vi "Fpga-FPGANic-Top.vi"() -> ()   [LabVIEW 2018]
uses:
  <instrlib>/_niInstr/Network/Ethernet/MAC/CLIP/v1/Resources.ctl
  <vilib>/Platform/TimedLoop/XDataNode/timing_clust.ctl
  <vilib>/Platform/TimedLoop/XDataNode/nitl_modes.ctl
  <vilib>/Platform/TimedLoop/XDataNode/wakeup.ctl
  States/FPGANic.Read.States.ctl
  <instrlib>/_niInstr/Network/Ethernet/MAC/Raw Stream/v1/niInstr Ethernet MAC Raw Stream v1.lvclass
  <instrlib>/_niInstr/Network/Ethernet/Utility/v1/FPGA/Network Data Stream.ctl
  States/FPGANic.Write.States.ctl
  <vilib>/rvi/Emulation/niFpgaSctlEmulationGetInTimedLoop.vi
  <vilib>/rvi/Emulation/niFpgaEmulationReportErrorSimple.vi
  <vilib>/rvi/Emulation/niFpgaGetClockAttributes.vi
  <vilib>/rvi/Emulation/niFpgaCriticalErrorInLSC.vi
  <vilib>/rvi/eio/common/nirviEmuTemplateMethod_errors.vi
  <vilib>/rvi/interface/RandomDataEmulation/niFpgaRandomDataHandleErrors.vi
  <vilib>/rvi/DataTransferAndStorage/Container/Common/niFpgaContainerGetUniqueNameForEmu.vi
  <vilib>/rvi/DataTransferAndStorage/Container/Common/niFpgaContainerSetEmuInfo.vi
  <vilib>/rvi/eio/common/nirviEmuReportErrorAndStop.vi
  <vilib>/rvi/DataTransferAndStorage/Container/Common/niFpgaContainerExecOnDevCompGetState.vi
  <vilib>/rvi/Emulation/niFpgaEmulationIsFPGAContextNoSignature.vi
  <vilib>/rvi/errors/niFpgaSetErrorForExecOnDevCompSimple.vi
  <vilib>/rvi/FIFO/Fifo_Resource/nirvififoEmulationSetSize.vi
  <vilib>/rvi/FIFO/Fifo_Resource/nirviFifoEmulationQueueMgr.vi
  <instcachedir>/0/nirviFifoEmulationQueueMgr_E5CAEC123FF24DC58D834DCA3CDAA9B5.lvgen/nirviFifoEmulationQueueMgr_E5CAEC123FF24DC58D834DCA3CDAA9B5_003.vi
  <vilib>/rvi/FIFO/Fifo_Resource/nirvififoEmulationDetermineInputValidOut.vi
  <vilib>/rvi/FIFO/Fifo_Resource/nirvififoEmulationCreateLock.vi
  <vilib>/rvi/Emulation/niFpgaProcessEmulError.vi
  <vilib>/rvi/FIFO/Fifo_Resource/nirvififoEmulationObtainLock.vi
  <vilib>/rvi/FIFO/Fifo_Resource/nirvififoEmulationReleaseLock.vi
  <vilib>/rvi/occurrence/nirviWaitOnOccurrenceBase.vi
  <vilib>/rvi/errors/nirviReportUnexpectedCaseInternalError.vi
  <vilib>/rvi/errors/nirviReportUnexpectedCaseInternalError (U32).vi
  <vilib>/Utility/error.llb/Clear Errors.vi
  <instrlib>/_niInstr/Network/Ethernet/MAC/Raw Stream/v1/Read End of Bad Frame.vi
  <instrlib>/_niInstr/Network/Ethernet/MAC/Raw Stream/v1/Read End of Good Frame.vi
  <instrlib>/_niInstr/Network/Ethernet/MAC/Raw Stream/v1/Read Data Stream.vi
  <instrlib>/_niInstr/Network/Ethernet/MAC/Raw Stream/v1/Write Data Stream.vi
  <instrlib>/_niInstr/Network/Ethernet/MAC/Raw Stream/v1/Write End of Good Frame.vi
  <vilib>/Platform/TimedLoop/XDataNode/XDataNode.xnode
  <vilib>/eio/EIONode/EIONode.xnode
  <vilib>/rvi/DataTransferAndStorage/Container/XNode/niFpgaContainer.xnode
  <vilib>/rvi/interface/RandomDataEmulation/nirviRandomDataFpgaReadWriteTemplate.vi
  <vilib>/rvi/LocalResourceManager/LocalResourceManager.xnode
  <vilib>/rvi/FIFO/Fifo_Resource/niFpgaFifoEmulationRefIn.vi
  <instrlib>/_niInstr/Network/Ethernet/MAC/CLIP/v1/niInstr Ethernet MAC - CLIP v1.lvclass
  <vilib>/Platform/TimedLoop/XDataNode/XDNodeRunTimeDep.lvlib
  <instrlib>/_niInstr/Network/Ethernet/Utility/v1/FPGA/niInstr Ethernet Utilities FPGA v1.lvlib
panel:
  in  "Zero-out":bool
  in  "Flip_in":bool
  in  "d_microblaze_i\\reset_rtl":bool=TRUE
  out "GPIO #1 out":u32
  in  "GPIO #1 in":u32
  in  "d_microblaze_i\\AXI_STR_RXD_3_tkeep":u8=15
  out "mgtrefclks_locked":bool
  out "mgtrefclks_valid":bool
  out "posc_complete":bool
  out "sPort0_Power_Good":bool
  out "sPort1_Power_Good":bool
  out "signal_detect_Port0":bool
  out "signal_detect_Port1":bool
  out "aBlockLockPort0":bool
  out "aBlockLockPort1":bool
  out "GPIO #2 out":u32
  in  "GPIO #2 in":u32
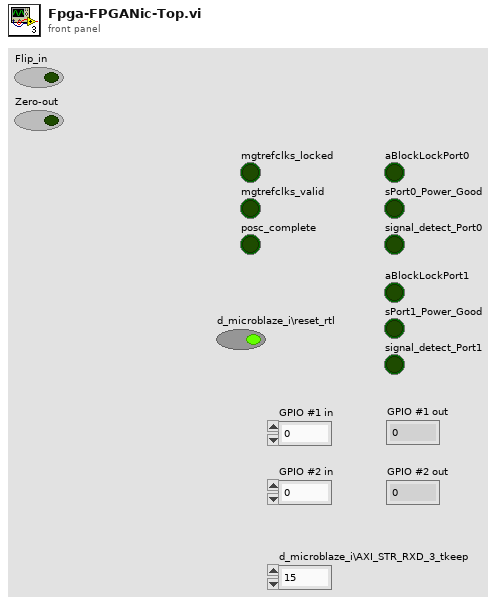
[diagram p1: front panel]
types:
  T1 = typedef "niInstr Ethernet MAC - CLIP v1.lvclass/Resources.ctl" = cluster{"RX":cluster{"TData":refnum<k21>, "TValid":refnum<k21>, "TKeep":refnum<k21>, "TLast":refnum<k21>, "TUser":refnum<k21>}, "TX":cluster{"TData":refnum<k21>, "TValid":refnum<k21>, "TKeep":refnum<k21>, "TLast":refnum<k21>, "TReady":refnum<k21>}, "Pause resources":cluster{"cPauseValuePort":refnum<k21>, "cPauseReqPort":refnum<k21>}, "MAC Clock":refnum<k21>}
  T2 = typedef "XDNodeRunTimeDep.lvlib/timing_clust.ctl" = cluster{"Expected End [f-1]":u64, "Actual End [f-1]":u64, "Finished Late? [f-1]":bool, "Expected End [i-1]":u64, "Actual End [i-1]":u64, "Finished Late? [i-1]":bool, "Expected Start [i]":u64, "Actual Start [i]":u64, "Expected Start [f]":u64, "Actual Start [f]":u64, "Source Name":string, "Structure Name":string, "Period":i64, "Deadline":i64, "Offset":i64, "Start":i64, "Priority":i32, "Timeout":i32, "Mode":T3, "Wakeup Reason":T4, "Error":errorcluster, "Source Type":string, "Secondary Source Type":string, "Global End Time":u64, "Global Start Time":u64, "Frame Duration":u64, "Iteration Duration":u64, "Assigned CPU":i32, "I/O Scan Engine Mode":u32}
  T3 = typedef "XDNodeRunTimeDep.lvlib/nitl_modes.ctl" = enum32{"No Change", "Process missed periods, maintain original phase", "Discard missed periods, maintain original phase", "Process missed periods, ignore original phase", "Discard missed periods, ignore original phase"}
  T4 = typedef "XDNodeRunTimeDep.lvlib/wakeup.ctl" = enum32{"Normal", "Aborted", "Asynchronous wakeup", "Timing source error", "Timed loop error", "Timeout"}
  T5 = typedef "niInstr Ethernet Utilities FPGA v1.lvlib/Network Data Stream.ctl" = cluster{"data":u8[], "data valid":bool, "byte enables":bool[]}
  T6 = cluster{"tdata[63:0]":u64, "tlast":bool, "tkeep[7:0]":bool[], "EndOfGoodFrame":bool, "EndOfBadFrame":bool}
  T7 = typedef "FPGANic.Write.States.ctl" = enum16{"Read-Top", "Read-Bottom"}
  T8 = typedef "FPGANic.Read.States.ctl" = enum16{"Read-Top", "Read-Bottom", "Append-Size"}
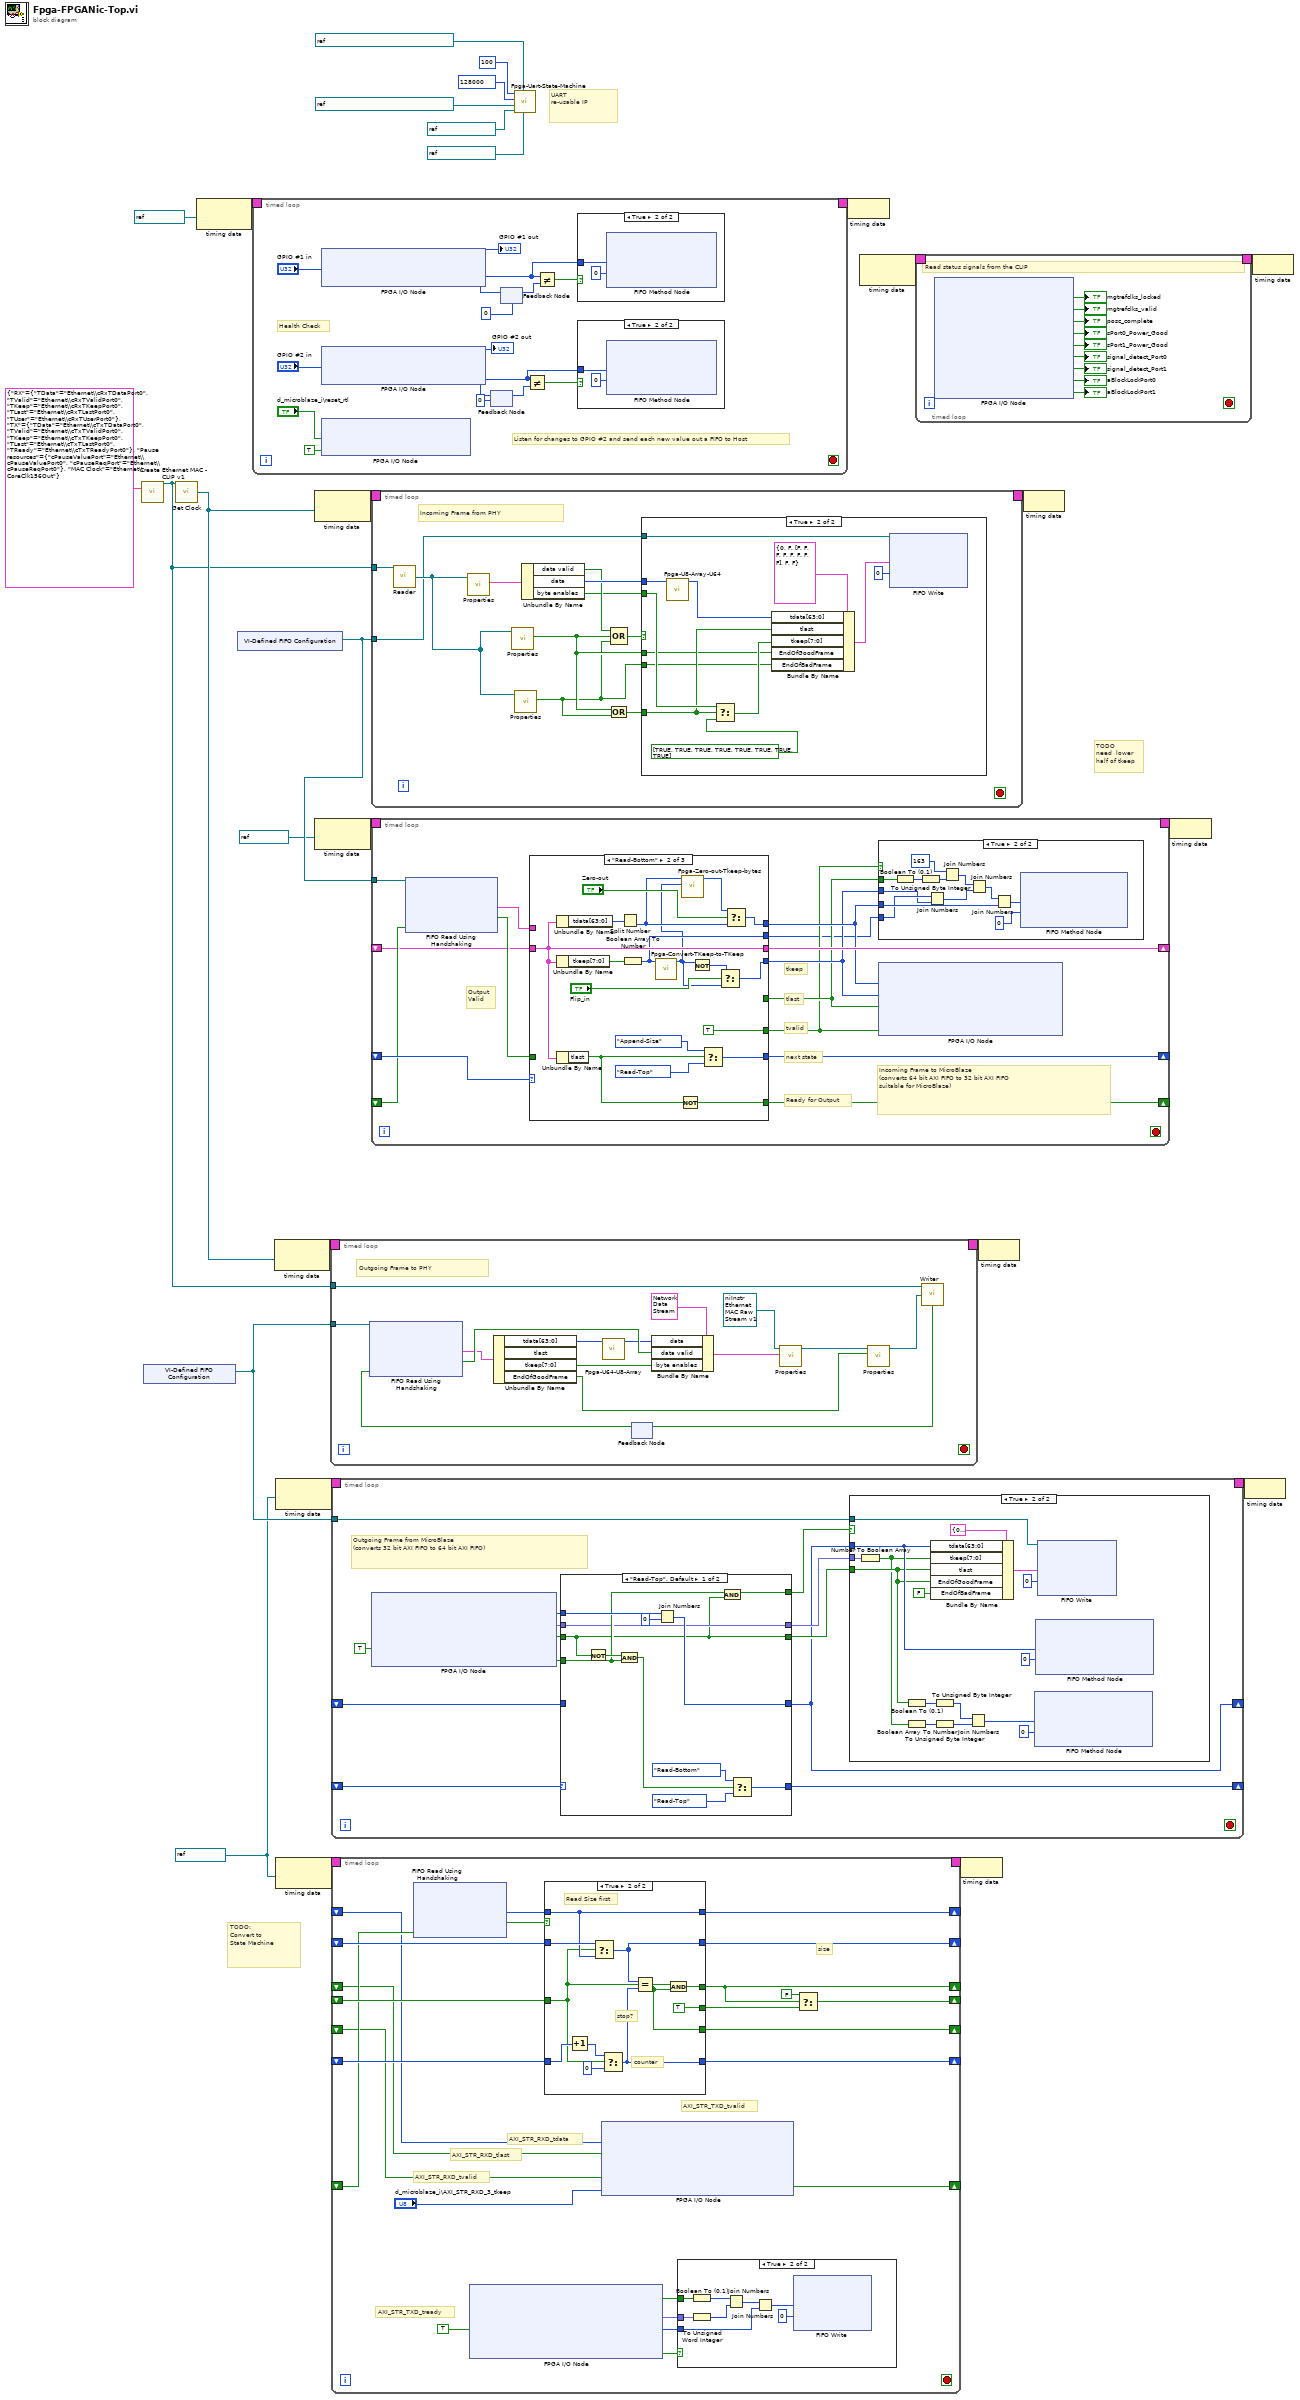
[diagram p0: block diagram]
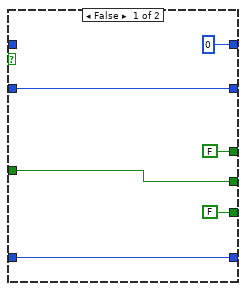
[diagram p3: hidden frame]
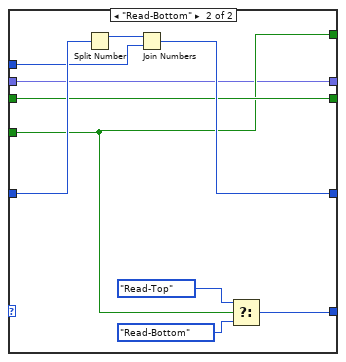
[diagram p4: hidden frame]
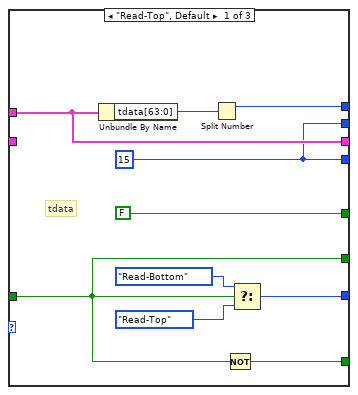
[diagram p6: hidden frame]
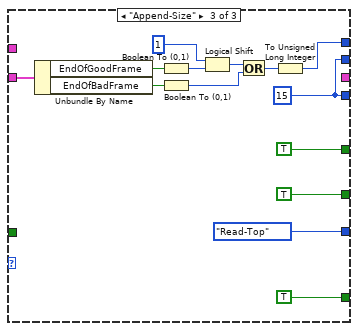
[diagram p7: hidden frame]
diagram:
  w5 = u32 128000 items=["110"=110, "300"=300, "1200"=1200, "2400"=2400, "4800"=4800, "9600"=9600, "19200"=19200, "38400"=38400, "57600"=57600, "115200"=115200, "128000"=128000, "230400"=230400, "460800"=460800, "921600"=921600] ("Baud Rate")
  w7 = refnum<k21> "100MHz" ("Source Name")
  # "UART\nre-usable IP"
  # "TODO:\nConvert to \nState Machine"
  # "TODO\nneed  lower\nhalf of tkeep"
  n1 = call <instrlib>:"Create Ethernet MAC - CLIP v1.vi"("Ethernet AXI4-S Resources"=T1 {"RX"={"TData"="Ethernet\\cRxTDataPort0", "TValid"="Ethernet\\cRxTValidPort0", "TKeep"="Ethernet\\cRxTKeepPort0", "TLast"="Ethernet\\cRxTLastPort0", "TUser"="Ethernet\\cRxTUserPort0"}, "TX"={"TData"="Ethernet\\cTxTDataPort0", "TValid"="Ethernet\\cTxTValidPort0", "TKeep"="Ethernet\\cTxTKeepPort0", "TLast"="Ethernet\\cTxTLastPort0", "TReady"="Ethernet\\cTxTReadyPort0"}, "Pause resources"={"cPauseValuePort"="Ethernet\\cPauseValuePort0", "cPauseReqPort"="Ethernet\\cPauseReqPort0"}, "MAC Clock"="Ethernet\\CoreClk156Out"}) -> ("niInstr Ethernet MAC - CLIP v1.lvclass out"=w17:refnum<class "niInstr Ethernet MAC - CLIP v1.lvclass">)  [unwired: 14 in]
  n2 = xnode "VI-Defined FIFO Configuration"() -> ("FIFO Out"=w10:refnum<k21>)
  n3 = call-dynamic "Get Clock.vi"("niInstr Ethernet MAC - CLIP v1.lvclass"=w17) -> ("MAC Clock"=w18:refnum<k21>)  [unwired: 14 in]
  n4 = node-c288(refnum<k21> "100MHz" ("Source Name")) -> (w28:T2)
  n5 = xnode "VI-Defined FIFO Configuration"() -> ("FIFO Out"=w14:refnum<k21>)
  n6 = timed-loop {
    timing: w28 -> [_]
    timing-out: [_] -> w27
    stop <- _ stop-if-true
    # "Health Check"
    # "Listen for changes to GPIO #2 and send each new value out a FIFO to Host"
    n7 = xnode "FPGA I/O Node"("UserRTL_microblaze\\gpio_rtl_tri_i"="GPIO #1 in") -> ("UserRTL_microblaze\\gpio_rtl_0_tri_o"=w32:u32)  [unwired: 2 in, 2 out]
    "GPIO #1 out" <- w32
    n8 = xnode "FPGA I/O Node"("UserRTL_microblaze\\gpio_rtl_1_tri_i"="GPIO #2 in") -> ("UserRTL_microblaze\\gpio_rtl_2_tri_o"=w34:u32)  [unwired: 2 in, 2 out]
    "GPIO #2 out" <- w34
    n9 = xnode "FPGA I/O Node"("UserRTL_microblaze\\reset_rtl"="d_microblaze_i\\reset_rtl", "UserRTL_microblaze\\uart_rtl_rxd"=TRUE ("d_microblaze_i\\uart_rtl_rxd")) -> ()  [unwired: 2 in, 2 out]
    n10 = feedback-in #1(w34) -> ()
    n11 = feedback #1(u32 0 ("d_microblaze_i\\gpio_rtl_2_tri_o")) -> (w39:u32)
    n12 = feedback #2(u32 0 ("d_microblaze_i\\gpio_rtl_0_tri_o")) -> (w37:u32)
    n13 = feedback-in #2(w32) -> ()
    n14 = Not Equal?(x=w34, y=w39) -> (x != y?=w36:bool)
    n15 = Not Equal?(x=w32, y=w37) -> (x != y?=w33:bool)
    n16 = case shown="True" w33 {
      tunnel: w32 -> [_ w42]
      frame False {
      }
      frame True {
        n17 = xnode ("FIFO Method Node")("Element"=w42, "Timeout"=0) -> ()  [unwired: 1 in, 2 out]
      }
    }
    n18 = case shown="True" w36 {
      tunnel: w34 -> [_ w44]
      frame False {
      }
      frame True {
        n19 = xnode ("FIFO Method Node")("Element"=w44, "Timeout"=0) -> ()  [unwired: 1 in, 2 out]
      }
    }
  }
  n20 = node-c288(w18) -> (w21:T2)
  n21 = node-c288(w7) -> (w12:T2)
  n22 = node-c288(w7) -> (w9:T2)
  n23 = node-c288(w18) -> (w25:T2)
  n24 = node-c288(refnum<k21> "100MHz" ("Source Name")) -> (w16:T2)
  n25 = timed-loop {
    timing: w21 -> [_]
    timing-out: [_] -> w20
    tunnel: w17 -> [w61]
    tunnel: w10 -> [w55]
    stop <- _ stop-if-true
    # "Outgoing Frame to PHY"
    n26 = feedback #3() -> (w54:bool)  [unwired: 1 in]
    n27 = xnode ("FIFO Read Using Handshaking")("Ready for Output"=w54, "FIFO In"=w55) -> ("Element"=w51:T6, "Output Valid"=w52:bool)  [unwired: 1 out]
    n28 = Unbundle By Name(w51) -> ("tdata[63:0]"=w48:u64, "tkeep[7:0]"=w49:bool[], "EndOfGoodFrame"=w50:bool)  [unwired: 1 out]
    n29 = call "Fpga-U64-U8-Array.vi"("U64 in"=w48) -> ("U8[] out"=w47:u8[])  [unwired: 10 in]
    n30 = Bundle By Name(cluster=T5 {"data"=[0, 0, 0, 0, 0, 0, 0, 0], "data valid"=FALSE, "byte enables"=[FALSE, FALSE, FALSE, FALSE, FALSE, FALSE, FALSE, FALSE]} ("Data Stream"), "data"=w47, "data valid"=w52, "byte enables"=w49) -> (w59:T5)
    n31 = call-poly <instrlib>:"Properties.vi"("Data Stream"=w59, "niInstr Ethernet MAC Data Stream v1 in"=refnum<class "niInstr Ethernet MAC Raw Stream v1.lvclass"> refnum) -> ("niInstr Ethernet MAC Data Stream v1 out"=w58:refnum<class "niInstr Ethernet MAC Raw Stream v1.lvclass">)  [unwired: 9 in]
    n32 = call-poly <instrlib>:"Properties.vi"("End of Good Frame"=w50, "niInstr Ethernet MAC Data Stream v1 in"=w58) -> ("niInstr Ethernet MAC Data Stream v1 out"=w56:refnum<class "niInstr Ethernet MAC Raw Stream v1.lvclass">)  [unwired: 9 in]
    n33 = call-dynamic "Writer.vi"("niInstr Ethernet MAC v1.lvclass"=w61, "niInstr Ethernet MAC Raw Stream v1.lvclass"=w56) -> ("ready for input?"=w53:bool)  [unwired: 12 in, 1 out]
    n34 = feedback-in #3(w53) -> ()
  }
  n35 = timed-loop {
    timing: w12 -> [_]
    timing-out: [_] -> w11
    tunnel: w10 -> [w75]
    shift-right: [w73] -> _
    shift-left: _ -> [w74]
    shift-right: [w64] -> _
    shift-left: _ -> [w69]
    stop <- _ stop-if-true
    # "Outgoing Frame from MicroBlaze\n(converts 32 bit AXI FIFO to 64 bit AXI FIFO)"
    n36 = xnode "FPGA I/O Node"("UserRTL_microblaze\\AXI_STR_TXD_tready"=TRUE ("d_microblaze_i\\AXI_STR_TXD_2_tready")) -> ("UserRTL_microblaze\\AXI_STR_TXD_tdata"=w72:u32, "UserRTL_microblaze\\AXI_STR_TXD_tkeep"=w66:fxp<+,4,4>, "UserRTL_microblaze\\AXI_STR_TXD_tlast"=w70:bool, "UserRTL_microblaze\\AXI_STR_TXD_tvalid"=w71:bool)  [unwired: 5 in, 5 out]
    n37 = case shown="\"Read-Top\", Default" w74 {
      tunnel: [w86 w96] -> w73
      tunnel: w72 -> [w85 w92]
      tunnel: w71 -> [w80 w90]
      tunnel: [w83 w95] -> w64
      tunnel: w70 -> [w77 w91]
      tunnel: [w77 w91] -> w68
      tunnel: w69 -> [_ w94]
      tunnel: [w78 w90] -> w67
      tunnel: w66 -> [w79 w89]
      tunnel: [w79 w89] -> w65
      frame "Read-Top", Default {
        n38 = Not(x=w77) -> (.not. x?=w82:bool)
        n39 = And(x=w82, y=w80) -> (x .and. y?=w81:bool)
        n40 = Join Numbers(hi=w85, lo=u32 0) -> ((hi.lo)=w83:u64)
        n41 = And(x=w80, y=w77) -> (x .and. y?=w78:bool)
        n42 = Select(t=FPGANic.Write.States."Read-Bottom" ("Enum"), s=w81, f=FPGANic.Write.States."Read-Top" ("Enum")) -> (s? t:f=w86:T7)
      }
      frame "Read-Bottom" {
        n43 = Split Number(x=w94) -> (hi(x)=w93:u32)  [unwired: 1 out]
        n44 = Join Numbers(hi=w93, lo=w92) -> ((hi.lo)=w95:u64)
        n45 = Select(t=FPGANic.Write.States."Read-Top" ("Enum"), s=w90, f=FPGANic.Write.States."Read-Bottom" ("Enum")) -> (s? t:f=w96:T7)
      }
    }
    n46 = case shown="True" w67 {
      tunnel: w75 -> [_ w114]
      tunnel: w64 -> [_ w109]
      tunnel: w68 -> [_ w100]
      tunnel: w65 -> [_ w113]
      frame False {
      }
      frame True {
        n47 = Number To Boolean Array(number=w113) -> (Boolean array=w99:bool[])
        n48 = Boolean To (0,1)(Boolean=w100) -> (0, 1=w105:i16)
        n49 = Boolean Array To Number(Boolean array=w99) -> (number=w103:u8)
        n50 = Bundle By Name(cluster=T6 {"tdata[63:0]"=0, "tlast"=FALSE, "tkeep[7:0]"=[FALSE, FALSE, FALSE, FALSE, FALSE, FALSE, FALSE, FALSE], "EndOfGoodFrame"=FALSE, "EndOfBadFrame"=FALSE} ("AXI4-Pins"), "tdata[63:0]"=w109, "tkeep[7:0]"=w99, "tlast"=w100, "EndOfGoodFrame"=w100, "EndOfBadFrame"=FALSE) -> (w111:T6)
        n51 = To Unsigned Byte Integer(number=w105) -> (unsigned 8bit integer=w104:u8)
        n52 = To Unsigned Byte Integer(number=w103) -> (unsigned 8bit integer=w102:u8)
        n53 = Join Numbers(hi=w104, lo=w102) -> ((hi.lo)=w106:u16)
        n54 = xnode ("FIFO Method Node")("Element"=w106, "Timeout"=0) -> ()  [unwired: 1 in, 2 out]
        n55 = xnode ("FIFO Method Node")("Element"=w109, "Timeout"=0) -> ()  [unwired: 1 in, 2 out]
        n56 = xnode ("FIFO Write")("Element"=w111, "Timeout"=0, "FIFO In"=w114) -> ()  [unwired: 2 out]
      }
    }
  }
  n57 = timed-loop {
    timing: w9 -> [_]
    timing-out: [_] -> w8
    shift-right: [w124] -> _
    shift-left: _ -> [w139]
    shift-right: [w136] -> _
    shift-left: _ -> [w138]
    shift-right: [w134] -> _
    shift-left: _ -> [w135]
    shift-right: [w122] -> _
    shift-left: _ -> [w129]
    shift-right: [w121] -> _
    shift-left: _ -> [w133]
    shift-right: [w132] -> _
    shift-left: _ -> [w131]
    shift-right: [w123] -> _
    shift-left: _ -> [w130]
    stop <- _ stop-if-true
    # "size"
    # "AXI_STR_TXD_tvalid"
    # "AXI_STR_TXD_tready"
    # "AXI_STR_RXD_tvalid"
    # "AXI_STR_RXD_tlast"
    # "AXI_STR_RXD_tdata"
    n58 = xnode ("FIFO Read Using Handshaking")("Ready for Output"=w133) -> ("Element"=w137:u64, "Output Valid"=w140:bool)  [unwired: 1 in, 1 out]
    n59 = xnode "FPGA I/O Node"("UserRTL_microblaze\\AXI_STR_TXD_1_tready"=TRUE ("d_microblaze\\AXI_STR_TXD_tready")) -> ("UserRTL_microblaze\\AXI_STR_TXD_1_tlast"=w118:bool, "UserRTL_microblaze\\AXI_STR_TXD_1_tkeep"=w117:fxp<+,4,4>, "UserRTL_microblaze\\AXI_STR_TXD_1_tdata"=w119:u32, "UserRTL_microblaze\\AXI_STR_TXD_1_tvalid"=w127:bool)  [unwired: 5 in, 5 out]
    n60 = case shown="True" w140 {
      tunnel: w139 -> [w153 w155]
      tunnel: [w153 TRUE ("Size\nRead?")] -> w125
      tunnel: w138 -> [w154 w165]
      tunnel: w137 -> [_ w160]
      tunnel: [w154 w159] -> w136
      tunnel: w135 -> [w152 w164]
      tunnel: [w152 w158] -> w134
      tunnel: [FALSE ("Size\nRead?") w155] -> w122
      tunnel: [u64 0 ("Element") w160] -> w132
      tunnel: [FALSE w156] -> w123
      frame False {
      }
      frame True {
        # "Read Size first"
        # "stop?"
        # "counter"
        n61 = Increment(x=w164) -> (x+1=w162:u64)
        n62 = Select(t=w165, s=w155, f=w160) -> (s? t:f=w159:u64)
        n63 = Select(t=w162, s=w155, f=u64 0) -> (s? t:f=w158:u64)
        n64 = Equal?(x=w159, y=w158) -> (x = y?=w157:bool)
        n65 = And(x=w157, y=w155) -> (x .and. y?=w156:bool)
      }
    }
    n66 = xnode "FPGA I/O Node"("UserRTL_microblaze\\AXI_STR_RXD_1_tdata"=w131, "UserRTL_microblaze\\AXI_STR_RXD_1_tlast"=w130, "UserRTL_microblaze\\AXI_STR_RXD_1_tvalid"=w129, "UserRTL_microblaze\\AXI_STR_RXD_1_tkeep"="d_microblaze_i\\AXI_STR_RXD_3_tkeep") -> ("UserRTL_microblaze\\AXI_STR_RXD_1_tready"=w121:bool)  [unwired: 5 in, 5 out]
    n67 = case shown="True" w127 {
      tunnel: w119 -> [_ w147]
      tunnel: w118 -> [_ w143]
      tunnel: w117 -> [_ w142]
      frame False {
      }
      frame True {
        n68 = Boolean To (0,1)(Boolean=w143) -> (0, 1=w144:i16)
        n69 = To Unsigned Word Integer(number=w142) -> (unsigned 16bit integer=w141:u16)
        n70 = Join Numbers(hi=w144, lo=w141) -> ((hi.lo)=w145:u32)
        n71 = Join Numbers(hi=w145, lo=w147) -> ((hi.lo)=w146:u64)
        n72 = xnode ("FIFO Write")("Element"=w146, "Timeout"=0) -> ()  [unwired: 1 in, 2 out]
      }
    }
    n73 = Select(t=FALSE, s=w123, f=w125) -> (s? t:f=w124:bool)
  }
  n74 = timed-loop {
    timing: w25 -> [_]
    timing-out: [_] -> w24
    tunnel: w17 -> [w178]
    tunnel: w14 -> [w174]
    stop <- _ stop-if-true
    # "Incoming Frame from PHY"
    n75 = call-dynamic "Reader.vi"("niInstr Ethernet MAC - CLIP v1.lvclass 2"=w178) -> ("niInstr Ethernet MAC Raw Stream v1.lvclass"=w175:refnum<class "niInstr Ethernet MAC Raw Stream v1.lvclass">)  [unwired: 13 in, 1 out]
    n76 = call-poly <instrlib>:"Properties.vi"("niInstr Ethernet MAC Data Stream v1 in"=w175) -> ("Data Stream"=w177:T5)  [unwired: 9 in, 1 out]
    n77 = call-poly <instrlib>:"Properties.vi"("niInstr Ethernet MAC Data Stream v1 in"=w175) -> ("End of Good Frame"=w169:bool)  [unwired: 9 in, 1 out]
    n78 = call-poly <instrlib>:"Properties.vi"("niInstr Ethernet MAC Data Stream v1 in"=w175) -> ("End of Bad Frame"=w168:bool)  [unwired: 9 in, 1 out]
    n79 = Unbundle By Name(w177) -> ("data valid"=w173:bool, "data"=w176:u8[], "byte enables"=w170:bool[])
    n80 = Or(x=w169, y=w168) -> (x .or. y?=w171:bool)
    n81 = Compound Arithmetic op=OR(w173, w169, w168) -> (w172:bool)
    n82 = case shown="True" w172 {
      tunnel: w176 -> [_ w188]
      tunnel: w174 -> [_ w189]
      tunnel: w171 -> [_ w182]
      tunnel: w170 -> [_ w183]
      tunnel: w169 -> [_ w181]
      tunnel: w168 -> [_ w180]
      frame False {
      }
      frame True {
        n83 = call "Fpga-U8-Array-U64.vi"("U8[] in"=w188) -> ("U64 out"=w185:u64)  [unwired: 10 in]
        n84 = Select(t=w183, s=w182, f=bool[] [TRUE, TRUE, TRUE, TRUE, TRUE, TRUE, TRUE, TRUE] ("s? t:f")) -> (s? t:f=w184:bool[])
        n85 = Bundle By Name(cluster=T6 {"tdata[63:0]"=0, "tlast"=FALSE, "tkeep[7:0]"=[FALSE, FALSE, FALSE, FALSE, FALSE, FALSE, FALSE, FALSE], "EndOfGoodFrame"=FALSE, "EndOfBadFrame"=FALSE} ("Element"), "tdata[63:0]"=w185, "tlast"=w182, "tkeep[7:0]"=w184, "EndOfGoodFrame"=w181, "EndOfBadFrame"=w180) -> (w186:T6)
        n86 = xnode ("FIFO Write")("Element"=w186, "Timeout"=0, "FIFO In"=w189) -> ()  [unwired: 2 out]
      }
    }
  }
  n87 = timed-loop {
    timing: w16 -> [_]
    timing-out: [_] -> w15
    tunnel: w14 -> [w206]
    shift-right: [w203] -> _
    shift-left: _ -> [w198]
    shift-right: [w202] -> _
    shift-left: _ -> [w201]
    shift-right: [w200] -> _
    shift-left: _ -> [w199]
    stop <- _ stop-if-true
    # "Incoming Frame to MicroBlaze\n(converts 64 bit AXI FIFO to 32 bit AXI FIFO\nsuitable for MicroBlaze)"
    # "Output\nValid"
    # "Ready for Output"
    # "next state"
    # "tkeep"
    # "tlast"
    # "tvalid"
    n88 = xnode ("FIFO Read Using Handshaking")("Ready for Output"=w199, "FIFO In"=w206) -> ("Element"=w204:T6, "Output Valid"=w205:bool)  [unwired: 1 out]
    n89 = case shown="\"Read-Bottom\"" w201 {
      tunnel: w205 -> [w209 _ _]
      tunnel: w204 -> [w210 _ _]
      tunnel: [w215 w222 w239] -> w197
      tunnel: [w212 w231 FPGANic.Read.States."Read-Top" ("Enum")] -> w202
      tunnel: [w209 TRUE ("Output Valid") TRUE ("Output Valid")] -> w194
      tunnel: [FALSE _ TRUE] -> w195
      tunnel: [w207 w223 w235] -> w196
      tunnel: [w210 w232 _] -> w203
      tunnel: [w208 w226 TRUE ("tlast")] -> w200
      tunnel: w198 -> [_ w232 w242]
      tunnel: [w207 w220 w235] -> w193
      frame "Read-Top", Default {
        w207 = u8 15 ("t")
        # "tdata"
        n90 = Unbundle By Name(w210) -> ("tdata[63:0]"=w216:u64)
        n91 = Split Number(x=w216) -> (hi(x)=w215:u32)  [unwired: 1 out]
        n92 = Not(x=w209) -> (.not. x?=w208:bool)
        n93 = Select(t=FPGANic.Read.States."Read-Bottom" ("Enum"), s=w209, f=FPGANic.Read.States."Read-Top" ("Enum")) -> (s? t:f=w212:T8)
      }
      frame "Read-Bottom" {
        n94 = Unbundle By Name(w232) -> ("tdata[63:0]"=w234:u64)
        n95 = Unbundle By Name(w232) -> ("tkeep[7:0]"=w233:bool[])
        n96 = Unbundle By Name(w232) -> ("tlast"=w228:bool)
        n97 = Split Number(x=w234) -> (lo(x)=w219:u32)  [unwired: 1 out]
        n98 = Boolean Array To Number(Boolean array=w233) -> (number=w220:u8)
        n99 = call "Fpga-Convert-TKeep-to-TKeep.vi"("tkeep (MAC)"=w220) -> ("tkeep (MicroBlaze)"=w217:u8)  [unwired: 10 in]
        n100 = Not(x=w228) -> (.not. x?=w226:bool)
        n101 = call "Fpga-Zero-out-Tkeep-bytes.vi"("tkeep (MAC)"=w217, "data_in"=w219) -> ("data_out"=w218:u32)  [unwired: 9 in]
        n102 = Not(x=w217) -> (.not. x?=w224:u8)
        n103 = Select(t=FPGANic.Read.States."Append-Size" ("Enum"), s=w228, f=FPGANic.Read.States."Read-Top" ("Enum")) -> (s? t:f=w231:T8)
        n104 = Select(t=w224, s="Flip_in", f=w217) -> (s? t:f=w223:u8)
        n105 = Select(t=w218, s="Zero-out", f=w219) -> (s? t:f=w222:u32)
      }
      frame "Append-Size" {
        w235 = u8 15 ("t")
        n106 = Unbundle By Name(w242) -> ("EndOfGoodFrame"=w241:bool, "EndOfBadFrame"=w240:bool)
        n107 = Boolean To (0,1)(Boolean=w241) -> (0, 1=w246:i16)
        n108 = Boolean To (0,1)(Boolean=w240) -> (0, 1=w243:i16)
        n109 = Logical Shift(y=i16 1, x=w246) -> (x << y=w244:i16)
        n110 = Or(x=w244, y=w243) -> (x .or. y?=w247:i16)
        n111 = To Unsigned Long Integer(number=w247) -> (unsigned 32bit integer=w239:u32)
      }
    }
    n112 = case shown="True" w194 {
      tunnel: w197 -> [_ w258]
      tunnel: w196 -> [_ w249]
      tunnel: w195 -> [_ w256]
      tunnel: w193 -> [_ w250]
      frame False {
      }
      frame True {
        n113 = Boolean To (0,1)(Boolean=w256) -> (0, 1=w255:i16)
        n114 = To Unsigned Byte Integer(number=w255) -> (unsigned 8bit integer=w254:u8)
        n115 = Join Numbers(hi=w250, lo=w249) -> ((hi.lo)=w251:u16)
        n116 = Join Numbers(hi=u8 163, lo=w254) -> ((hi.lo)=w253:u16)
        n117 = Join Numbers(hi=w253, lo=w251) -> ((hi.lo)=w257:u32)
        n118 = Join Numbers(hi=w257, lo=w258) -> ((hi.lo)=w259:u64)
        n119 = xnode ("FIFO Method Node")("Element"=w259, "Timeout"=0) -> ()  [unwired: 1 in, 2 out]
      }
    }
    n120 = xnode "FPGA I/O Node"("UserRTL_microblaze\\AXI_STR_RXD_tdata"=w197, "UserRTL_microblaze\\AXI_STR_RXD_tkeep"=w196, "UserRTL_microblaze\\AXI_STR_RXD_tlast"=w195, "UserRTL_microblaze\\AXI_STR_RXD_tvalid"=w194) -> ()  [unwired: 5 in, 6 out]
  }
  n121 = call "Fpga-Uart-State-Machine.vi"("TX FIFO In"=refnum<k21> "HT-UART_TX", "RXD Pin In"=refnum<k21> "UserRTL_microblaze\\uart_rtl_rxd", "RX FIFO In"=refnum<k21> "TH-UART_RX", "TXD Pin In"=refnum<k21> "UserRTL_microblaze\\uart_rtl_txd", "Baud Rate"=w5, "FPGA Clock Rate (MHz)"=u32 100) -> ()  [unwired: 6 in]
  n122 = node-c288(w27) -> ()
  n123 = node-c288() -> (w23:T2)  [unwired: 1 in]
  n124 = timed-loop {
    timing: w23 -> [_]
    timing-out: [_] -> w22
    stop <- _ stop-if-true
    # "Read status signals from the CLIP"
    n125 = xnode "FPGA I/O Node"() -> ("Ethernet\\MgtRefClks_Locked"=→"mgtrefclks_locked":bool, "Ethernet\\MgtRefClks_Valid"=→"mgtrefclks_valid":bool, "Ethernet\\POSC_Complete"=→"posc_complete":bool, "Ethernet\\sPort0_Power_Good"=→"sPort0_Power_Good":bool, "Ethernet\\sPort1_Power_Good"=→"sPort1_Power_Good":bool, "Ethernet\\signal_detect_Port0"=→"signal_detect_Port0":bool, "Ethernet\\signal_detect_Port1"=→"signal_detect_Port1":bool, "Ethernet\\aBlockLockPort0"=→"aBlockLockPort0":bool, "Ethernet\\aBlockLockPort1"=→"aBlockLockPort1":bool)  [unwired: 9 in, 9 out]
  }
  n126 = node-c288(w8) -> ()
  n127 = node-c288(w20) -> ()
  n128 = node-c288(w24) -> ()
  n129 = node-c288(w15) -> ()
  n130 = node-c288(w11) -> ()
  n131 = node-c288(w22) -> ()
